vi "RSNRPZ Configure Reflection Gamma Corr.vi"(7 "Phase (0.0 deg)":dbl format="%^.3e", 8 "error in (no error)":errorcluster, 9 "Magnitude (0.0)":dbl format="%^.3e", 10 "Channel (1)":i32=1, 11 "VISA session":refnum<visa-resource-name> caption="VISA resource name") -> (0 "error out":errorcluster, 3 "dup VISA session":refnum<visa-resource-name> caption="VISA resource name")   [LabVIEW 2010]
doc: "This VI sets the parameters of the compensation of the load distortion at the signal output.\n\nNote(s):\n\n(1) This VI is available only for sensors NRP-Z27 and NRP-Z37\n\nRemote-control command(s):\nSENS:RGAM\nSENS:RGAM:PHAS"
uses:
  rsnrpz_32.dll
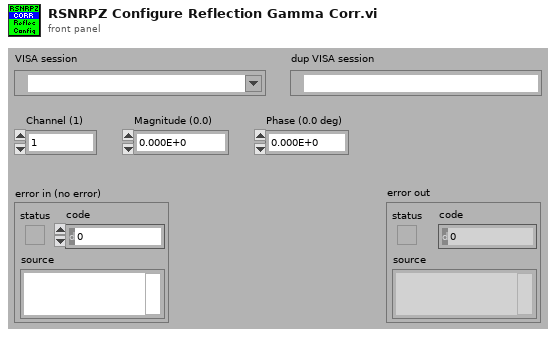
[diagram p1: front panel]
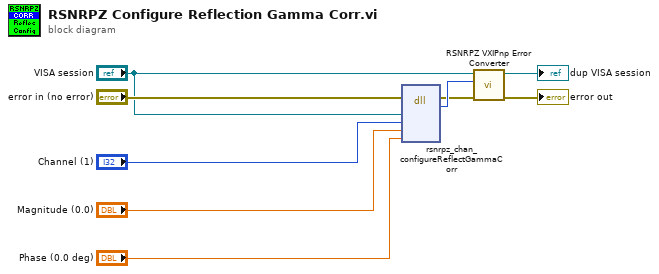
[diagram p0: block diagram]
diagram:
  n1 = dll-call lib="rsnrpz_32.dll" fn="rsnrpz_chan_configureReflectGammaCorr"(error in="error in (no error)", "Instrument Handle"="VISA session", "Channel"="Channel (1)", "Magnitude"="Magnitude (0.0)", "Phase"="Phase (0.0 deg)") -> (error out=w5:errorcluster, "Status"=w9:i32)  [unwired: 6 in, 1 out]
  n2 = call <instrlib>:"RSNRPZ VXIPnp Error Converter.vi"("error in"=w5, "VXIPnp error code"=w9, "VISA session"="VISA session") -> ("error out"=→"error out":errorcluster, "dup VISA session"=→"dup VISA session":refnum<visa-resource-name>)  [unwired: 7 in]
